vi "Set Wavelength.vi"(8 "error in (no error)":errorcluster, 10 "Wavelength (nm)":dbl, 11 "Simulated in":refnum<class "Simulated.lvclass">) -> (0 "error out":errorcluster, 2 "Wavelength (nm) out":dbl, 3 "Simulated out":refnum<class "Simulated.lvclass">)   [LabVIEW 2019, in "Simulated.lvclass"]
uses:
  Simulated.lvclass
  Simulated.lvclass/Simulated.ctl
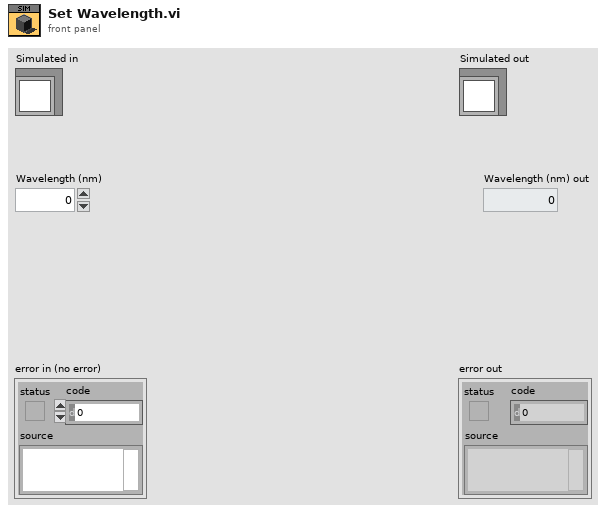
[diagram p1: front panel]
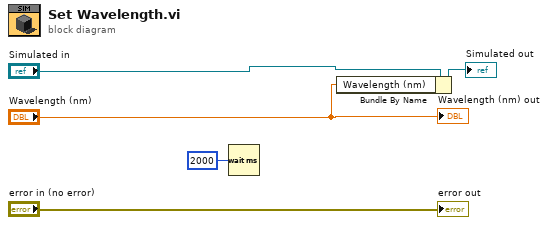
[diagram p0: block diagram]
diagram:
  n1 = Wait (ms)(milliseconds to wait=u32 2000) -> ()  [unwired: 1 out]
  n2 = Bundle By Name(cluster="Simulated in", "Wavelength (nm)"="Wavelength (nm)") -> (→"Simulated out":refnum<class "Simulated.lvclass">)
  "error out" <- "error in (no error)"
  "Wavelength (nm) out" <- "Wavelength (nm)"
